vi "Subtract float (multiple).vi"(8 "error in (no error)":errorcluster, 9 "y (0)":dbl, 10 "x (0)":dbl, 11 "XY-data":cluster{"X-array":dbl[], "Y-array":dbl[]}[](array[cluster]) {"Y-array" format="%.2p"; "X-array" format="%.2p"}) -> (0 "error out":errorcluster, 3 "XY-data out":cluster{"X-array":dbl[], "Y-array":dbl[]}[](array[cluster]) {"Y-array" format="%.2p"; "X-array" format="%.2p"})   [LabVIEW 2019, in "xy_utilities.lvlib"]
doc: "Subtract <b>x</b> from the x array of <b>XY-data</b>\nSubtract <b>y</b> from the y array of <b>XY-data</b>\n\nWire data to the data input to determine the polymorphic instance to use or manually select the instance."
uses:
  xy_utilities.lvlib
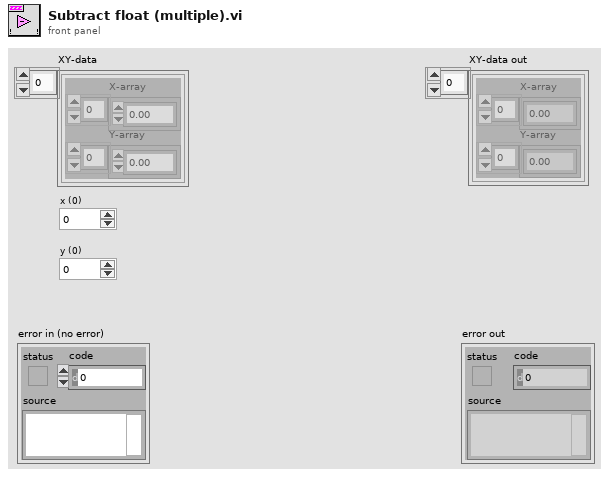
[diagram p1: front panel]
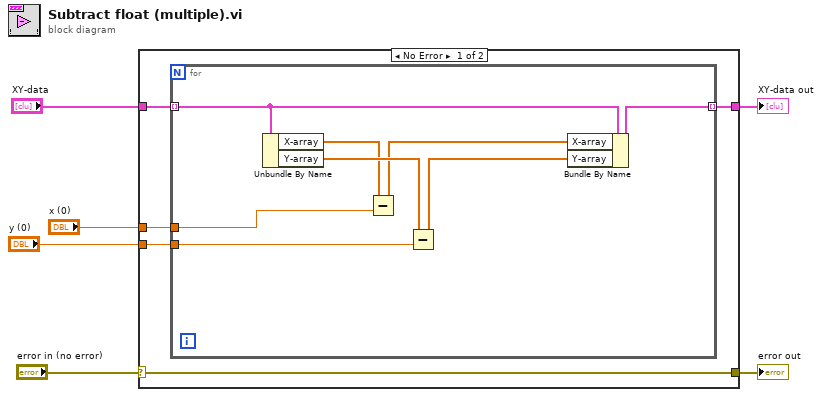
[diagram p0: block diagram]
diagram:
  n1 = case shown="No Error" "error in (no error)" {
    selector: "error in (no error)" -> [w11 w21]
    tunnel: [w11 w21] -> w5
    tunnel: "XY-data" -> [w10 w20]
    tunnel: [w9 w20] -> w3
    tunnel: "y (0)" -> [w8 _]
    tunnel: "x (0)" -> [w7 _]
    frame No Error {
      n2 = for {
        tunnel: w10 -> [w19] mode=indexing
        tunnel: [w18] -> w9 mode=indexing
        tunnel: w8 -> [w17]
        tunnel: w7 -> [w12]
        n3 = Unbundle By Name(w19) -> ("X-array"=w14:dbl[], "Y-array"=w16:dbl[])
        n4 = Subtract(x=w14, y=w12) -> (x-y=w13:dbl[])
        n5 = Subtract(x=w16, y=w17) -> (x-y=w15:dbl[])
        n6 = Bundle By Name(cluster=w19, "X-array"=w13, "Y-array"=w15) -> (w18:cluster{"X-array":dbl[], "Y-array":dbl[]})
      }
    }
    frame Error {
    }
  }
  "error out" <- w5
  "XY-data out" <- w3
